vi "Receive 10-100.vi"() -> ()   [LabVIEW 2015]
panel:
  out "100 byte":i32[][](array[numeric])
  out "Counter 100":i32
  out "Time":u32
  out "10 byte":u64[](array[numeric])
  out "Counter 10":i32
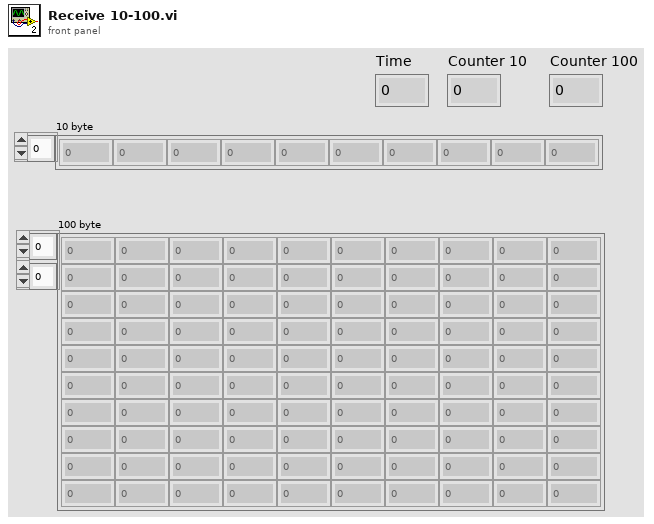
[diagram p1: front panel]
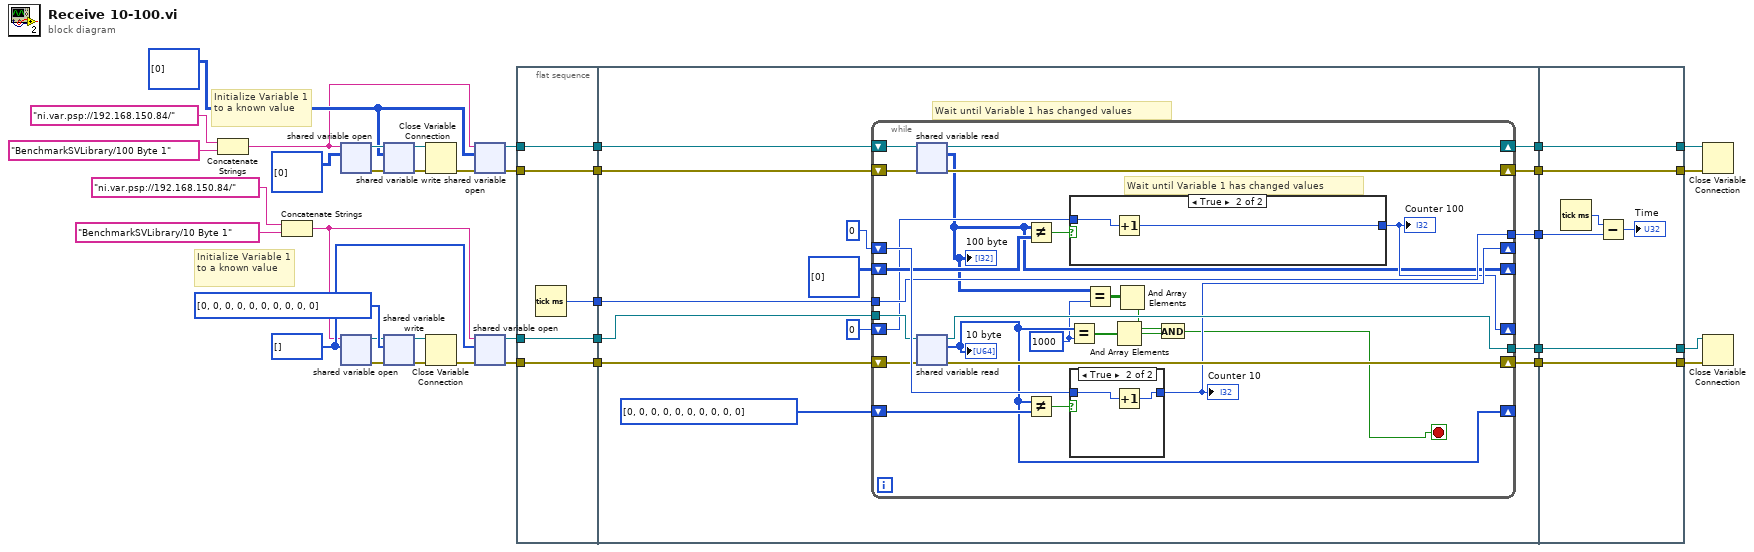
[diagram p0: block diagram]
diagram:
  w10 = i32[][] [[0]] ("1000 Byte 3")
  w24 = u64[] [] ("appended array")
  # "Initialize Variable 1 to a known value"
  # "Initialize Variable 1 to a known value"
  n1 = Concatenate Strings("ni.var.psp://192.168.150.84/" ("string"), "BenchmarkSVLibrary/100 Byte 1") -> (w9:string)
  n2 = Concatenate Strings("ni.var.psp://192.168.150.84/" ("string"), "BenchmarkSVLibrary/10 Byte 1") -> (w23:string)
  n3 = shared-variable-open(w9, i32[][] [[0]] ("appended array")) -> (w17:refnum<k21>, w15:errorcluster)  [unwired: 2 in]
  n4 = shared-variable-open(w23, w24) -> (w21:refnum<k21>, w26:errorcluster)  [unwired: 2 in]
  n5 = shared-variable-write(w17, w15, w10) -> (w16:refnum<k21>, w14:errorcluster)
  n6 = shared-variable-write(w21, w26, u64[] [0, 0, 0, 0, 0, 0, 0, 0, 0, 0] ("appended array")) -> (w20:refnum<k21>, w25:errorcluster)
  n7 = Close Variable Connection(8:w14, 11:w16) -> (0:w11:errorcluster)
  n8 = Close Variable Connection(8:w25, 11:w20) -> (0:w19:errorcluster)
  n9 = shared-variable-open(w9, w11, w10) -> (w4:refnum<k21>, w7:errorcluster)  [unwired: 1 in]
  n10 = shared-variable-open(w23, w19, w24) -> (w29:refnum<k21>, w30:errorcluster)  [unwired: 1 in]
  n11 = flat-sequence {
    tunnel: w29 -> [w42]
    tunnel: w30 -> [w43]
    tunnel: [w43] -> w38
    tunnel: [w42] -> w37
    tunnel: [w41] -> w36
    tunnel: [w40] -> w8
    tunnel: w7 -> [w40]
    tunnel: [w39] -> w5
    tunnel: w4 -> [w39]
    tunnel: [w54] -> w35
    tunnel: [w53] -> w34
    tunnel: [w51] -> w33
    tunnel: w38 -> [w57]
    tunnel: w37 -> [w56]
    tunnel: w36 -> [w52]
    tunnel: w8 -> [w47]
    tunnel: [w46] -> w6
    tunnel: w5 -> [w45]
    tunnel: [w44] -> w3
    tunnel: w35 -> [w91]
    tunnel: w34 -> [w92]
    tunnel: w33 -> [w93]
    tunnel: [w92] -> w28
    tunnel: [w91] -> w27
    tunnel: [w90] -> w2
    tunnel: w6 -> [w90]
    tunnel: [w89] -> w1
    tunnel: w3 -> [w89]
    frame #0 {
      n12 = Tick Count (ms)() -> (millisecond timer value=w41:u32)
    }
    frame #1 {
      # "Wait until Variable 1 has changed values"
      n13 = while {
        shift-right: [w73] -> _
        shift-left: u64[] [0, 0, 0, 0, 0, 0, 0, 0, 0, 0] ("appended array") -> [w82]
        shift-right: [w80] -> w54
        shift-left: w57 -> [w78]
        shift-right: [w74] -> _
        shift-left: 0 -> [w81]
        tunnel: w56 -> [w79]
        tunnel: [w77] -> w53
        tunnel: [w75] -> w51
        tunnel: w52 -> [w75]
        shift-right: [w62] -> _
        shift-left: i32[][] [[0]] ("1000 Byte 3") -> [w70]
        shift-right: [w68] -> _
        shift-left: 0 -> [w69]
        shift-right: [w66] -> w46
        shift-left: w47 -> [w67]
        shift-right: [w64] -> w44
        shift-left: w45 -> [w65]
        stop <- w58 stop-if-true
        w61 = 1000 ("y")
        # "Wait until Variable 1 has changed values"
        n14 = shared-variable-read(w65, w67) -> (w64:refnum<k21>, w66:errorcluster, w62:i32[][])  [unwired: 1 out]
        "100 byte" <- w62
        n15 = shared-variable-read(w79, w78) -> (w77:refnum<k21>, w80:errorcluster, w73:u64[])  [unwired: 1 out]
        "10 byte" <- w73
        n16 = Not Equal?(x=w62, y=w70) -> (x != y?=w71:bool)
        n17 = Not Equal?(x=w73, y=w82) -> (x != y?=w76:bool)
        n18 = Equal?(x=w73, y=w61) -> (x = y?=w72:bool[])
        n19 = case shown="True" w71 {
          tunnel: w69 -> [w83 w85]
          tunnel: [w83 w84] -> w68
          frame False {
          }
          frame True {
            n20 = Increment(x=w85) -> (x+1=w84:i32)
          }
        }
        "Counter 100" <- w68
        n21 = case shown="True" w76 {
          tunnel: w81 -> [w86 w88]
          tunnel: [w86 w87] -> w74
          frame False {
          }
          frame True {
            n22 = Increment(x=w88) -> (x+1=w87:i32)
          }
        }
        "Counter 10" <- w74
        n23 = Equal?(x=w62, y=w61) -> (x = y?=w63:bool[][])
        n24 = And Array Elements(Boolean array=w72) -> (logical AND=w60:bool)
        n25 = And Array Elements(Boolean array=w63) -> (logical AND=w59:bool)
        n26 = And(x=w59, y=w60) -> (x .and. y?=w58:bool)
      }
    }
    frame #2 {
      n27 = Tick Count (ms)() -> (millisecond timer value=w95:u32)
      n28 = Subtract(x=w95, y=w93) -> (x-y=→"Time":u32)
    }
  }
  n29 = Close Variable Connection(8:w2, 11:w1) -> ()  [unwired: 1 out]
  n30 = Close Variable Connection(8:w27, 11:w28) -> ()  [unwired: 1 out]
